vi "autonomousbarrystyle.vi"() -> ()   [LabVIEW 2010, in "Rampage.lvrbt"]
uses:
  Rampage.lvrbt
  <vilib>/NXT/Dual Mode Library/Waits/Wait_Num(msec).vi
  <vilib>/NXT/Block Support/NXT_InputPort.ctl
  <vilib>/NXT/HiTechnic/HiTechnic Controls/HiTechnic Port.ctl
  <vilib>/NXT/Subs/MotorOutput.ctl
  <vilib>/NXT/Subs/MotorXNode.DC Motor Type.ctl
  <vilib>/NXT/Subs/MotorXNode.2DCMotor.ctl
  <vilib>/NXT/Subs/LVHSConnector.ctl
  <vilib>/NXT/NXTIO Xnodes/NXTIONodeSubVIs/TETRIX IO Move DC Motors.vi
  <vilib>/NXT/NXTIO Xnodes/NXTIOXNode/NXTIO.xnode
  <vilib>/NXT/Dual Mode Library/Motors/MotorOn.vi
  <vilib>/NXT/Dual Mode Library/prims/inRangeAndCoerce/inRangeAndCoerce_int.vi
  <vilib>/NXT/NXTIO Xnodes/NXTIONodeSubVIs/TETRIX IO Stop DC Motors.vi
  <vilib>/NXT/NXTIO Xnodes/AddressXNode/NXTIOAddress.xnode
  <vilib>/NXT/Dual Mode Library/Sensors/Sonar_cm.vi
  <vilib>/NXT/Dual Mode Library/Waits/Wait_Num.vi
panel:
  out "Enabled":bool
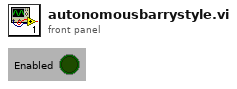
[diagram p1: front panel]
types:
  T1 = typedef "LVHSConnector.ctl" = cluster{"Hardware":string, "Flattened String":string}
  T2 = typedef "MotorOutput.ctl" = u8
  T3 = typedef "MotorXNode.DC Motor Type.ctl" = enum16{"DC Motor"}
  T4 = cluster{"DC Motor":T3, "Address":i16, "Address":i16}
  T5 = typedef "HiTechnic Port.ctl" = cluster{"Port":T6, "MUX Port":u8}
  T6 = typedef "NXT_InputPort.ctl" = u8
  T7 = cluster{"Direction (0-9)":i16, "Signal Strength (Array)":u8[]}
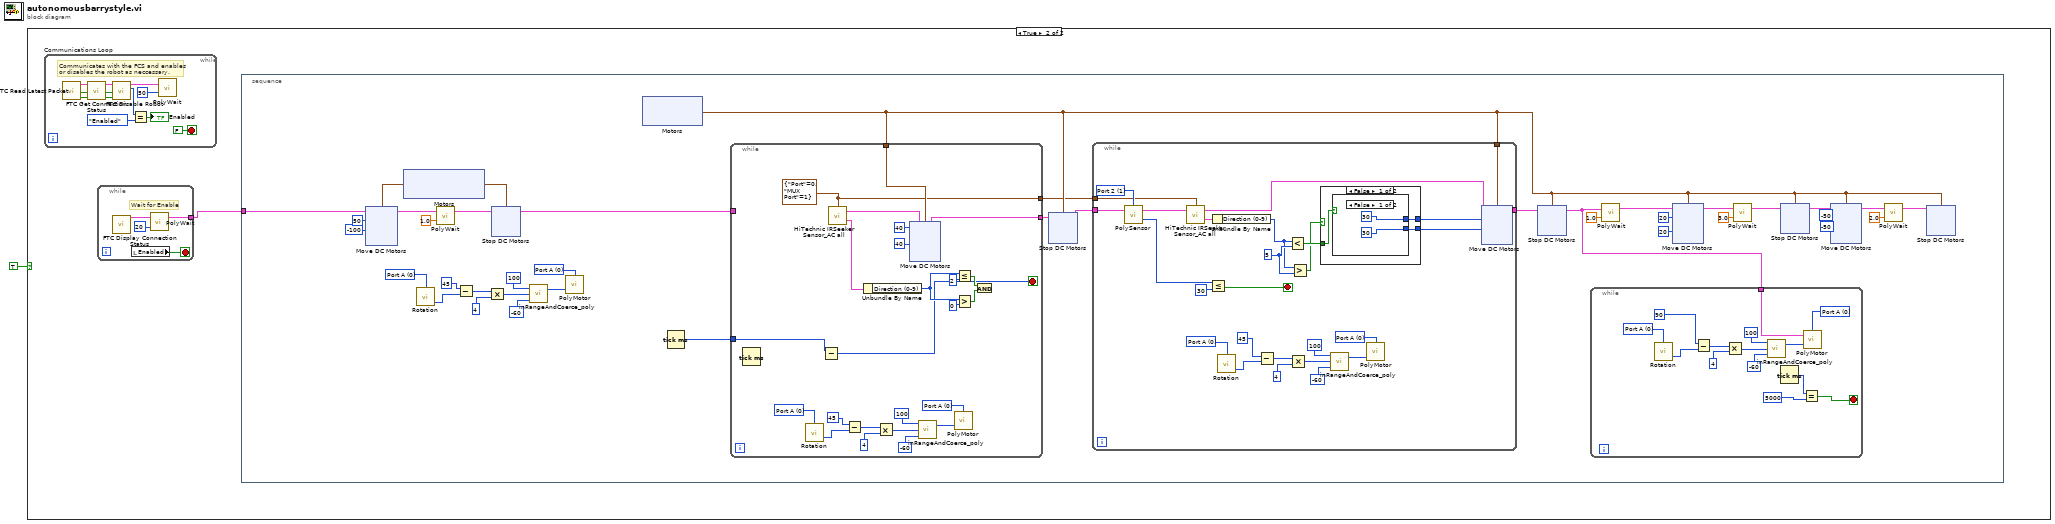
[diagram p0: block diagram]
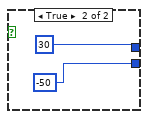
[diagram p3: hidden frame]
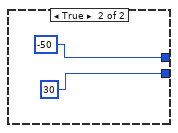
[diagram p4: hidden frame]
diagram:
  n1 = case shown="True" TRUE {
    frame False {
    }
    frame True {
      n2 = while "Communications Loop" {
        stop <- FALSE stop-if-true
        # "Communicates with the FCS and enables \nor disables the robot as neccessary."
        n3 = call <vilib>:"FTC Read Latest Packet.vi"() -> ("Packet Received?"=w216:bool, "Stopped?"=w215:bool, "NXT"=w218:T1)  [unwired: 6 in, 3 out]
        n4 = call <vilib>:"FTC Get Connection Status.vi"("Packet Received?"=w216, "Stopped?"=w215, "NXT"=w218) -> ("Online?"=w207:bool, "Stopped?"=w208:bool, "NXT"=w217:T1)  [unwired: 5 in]
        n5 = call <vilib>:"FTC Disable Robot.vi"("Online?"=w207, "Stopped?"=w208, "NXT"=w217) -> ("Enabled?"=w211:enum16{"Disabled", "Enabled"}, "NXT"=w213:T1)  [unwired: 3 in]
        n6 = Equal?(x=w211, y=enum16{"Disabled", "Enabled"}."Enabled") -> (x = y?=→"Enabled":bool)
        n7 = call-poly <vilib>:"PolyWait.vi"("Time (100 msec)"=u32 50 ("Time (msec)"), "NXT"=w213) -> ()  [unwired: 2 in, 1 out]
      }
      n8 = while {
        tunnel: [w204] -> w2
        stop <- w205 stop-if-true
        # "Wait for Enable"
        n9 = call <vilib>:"FTC Display Connection Status.vi"() -> ("NXT"=w203:T1)  [unwired: 11 in]
        n10 = local read "Enabled"() -> (w205:bool)
        n11 = call-poly <vilib>:"PolyWait.vi"("Time (100 msec)"=u32 20 ("Time (msec)"), "NXT"=w203) -> ("NXT"=w204:T1)  [unwired: 2 in]
      }
      n12 = stacked-sequence {
        tunnel: w2 -> [w5]
        frame #0 {
          w32 = T2 0 items=["Port A"=0, "Port B"=1, "Port C"=2, "Ports A & B"=4, "Ports A & C"=5, "Ports B & C"=6, "All Ports"=3] ("Output Port (All Ports)")
          w30 = u8 0 items=["Port A", "Port B", "Port C"] ("Port (Port A)")
          n13 = xnode "Motors"() -> ("DC Motor"=w40:T4)
          n14 = xnode "Move DC Motors"("Power/Speed 1"=i8 50, "Motors"=w40, "NXT"=w5, "Power/Speed 2"=i8 -100) -> ("NXT"=w38:T1)
          n15 = call <vilib>:"Rotation.vi"("Port (Port A)"=w30) -> ("Angle of Rotation"=w33:i32)  [unwired: 2 in, 1 out]
          n16 = call-poly <vilib>:"PolyWait.vi"("Time (1 sec)"=sgl 1.0, "NXT"=w38) -> ("NXT"=w35:T1)  [unwired: 2 in]
          n17 = Subtract(x=45 ("Claw\nPosition"), y=w33) -> (x-y=w31:i32)
          n18 = Multiply(x=w31, y=4) -> (x*y=w29:i32)
          n19 = xnode "Stop DC Motors"("Motors"=w40, "NXT"=w35) -> ("NXT"=w21:T1)
          n20 = call-poly <vilib>:"inRangeAndCoerce_poly.vi"("lower limit"=-60, "x"=w29, "upper limit"=100) -> ("coerced(x)"=w26:i32)  [unwired: 1 out]
          n21 = call-poly <vilib>:"PolyMotor.vi"("Power (75)"=w26, "Output Port (All Ports)"=w32) -> ()  [unwired: 2 in, 1 out]
          n22 = xnode "Motors"() -> ("DC Motor"=w23:T4)
          n23 = Tick Count (ms)() -> (millisecond timer value=w3:u32)
          n24 = while {
            tunnel: [w191] -> w9
            tunnel: w23 -> [w188]
            tunnel: [w175] -> w4
            tunnel: w21 -> [_]
            tunnel: w3 -> [w170]
            stop <- w169 stop-if-true
            w180 = T2 0 items=["Port A"=0, "Port B"=1, "Port C"=2, "Ports A & B"=4, "Ports A & C"=5, "Ports B & C"=6, "All Ports"=3] ("Output Port (All Ports)")
            w182 = u8 0 items=["Port A", "Port B", "Port C"] ("Port (Port A)")
            w175 = T5 {"Port"=0, "MUX Port"=1} ("Port/MUX")
            n25 = Tick Count (ms)() -> ()  [unwired: 1 out]
            n26 = call <vilib>:"Rotation.vi"("Port (Port A)"=w182) -> ("Angle of Rotation"=w179:i32)  [unwired: 2 in, 1 out]
            n27 = Subtract(x=w170) -> (y=w168:u32, x-y=w169:u32)
            n28 = call <vilib>:"HiTechnic IRSeeker Sensor_AC all.vi"("Port/MUX"=w175) -> ("All Info"=w176:T7, "NXT"=w192:T1)  [unwired: 2 in]
            n29 = Subtract(x=45 ("Claw\nPosition"), y=w179) -> (x-y=w181:i32)
            n30 = Unbundle By Name(w176) -> ("Direction (0-9)"=w173:i16)
            n31 = Multiply(x=w181, y=4) -> (x*y=w183:i32)
            n32 = xnode "Move DC Motors"("Power/Speed 2"=i8 40, "Power/Speed 1"=i8 40, "Motors"=w188, "NXT"=w192) -> ("NXT"=w191:T1)
            n33 = call-poly <vilib>:"inRangeAndCoerce_poly.vi"("lower limit"=-60, "x"=w183, "upper limit"=100) -> ("coerced(x)"=w186:i32)  [unwired: 1 out]
            n34 = call-poly <vilib>:"PolyMotor.vi"("Power (75)"=w186, "Output Port (All Ports)"=w180) -> ()  [unwired: 2 in, 1 out]
            n35 = Less Or Equal?(x=w173, y=i16 2) -> (x <= y?=w172:bool)
            n36 = Greater?(x=w173, y=i16 0) -> (0:w171:bool)
            n37 = And(x=w172, y=w171) -> ()  [unwired: 1 out]
          }
          n38 = xnode "Stop DC Motors"("Motors"=w23, "NXT"=w9) -> ("NXT"=w24:T1)
          n39 = while {
            tunnel: [w139] -> w8
            tunnel: w23 -> [w138]
            tunnel: w24 -> [w116]
            tunnel: w4 -> [w114]
            stop <- w115 stop-if-true
            w119 = T2 0 items=["Port A"=0, "Port B"=1, "Port C"=2, "Ports A & B"=4, "Ports A & C"=5, "Ports B & C"=6, "All Ports"=3] ("Output Port (All Ports)")
            w121 = u8 0 items=["Port A", "Port B", "Port C"] ("Port (Port A)")
            w130 = i16 5 ("y")
            w136 = T6 1 items=["Port 1", "Port 2", "Port 3", "Port 4"] ("Port (Port 4)")
            n40 = call-poly <vilib>:"PolySensor.vi"("NXT"=w116, "Port (Port 4)"=w136) -> ("Distance (cm)"=w137:i16, "NXT"=w135:T1)  [unwired: 1 in]
            n41 = call <vilib>:"HiTechnic IRSeeker Sensor_AC all.vi"("NXT"=w135, "Port/MUX"=w114) -> ("All Info"=w134:T7, "NXT"=w133:T1)  [unwired: 1 in]
            n42 = Less Or Equal?(x=w137, y=i16 30) -> (x <= y?=w115:bool)
            n43 = Unbundle By Name(w134) -> ("Direction (0-9)"=w129:i16)
            n44 = call <vilib>:"Rotation.vi"("Port (Port A)"=w121) -> ("Angle of Rotation"=w118:i32)  [unwired: 2 in, 1 out]
            n45 = Subtract(x=45 ("Claw\nPosition"), y=w118) -> (x-y=w120:i32)
            n46 = Less?(x=w129, y=w130) -> (x < y?=w128:bool)
            n47 = Multiply(x=w120, y=4) -> (x*y=w122:i32)
            n48 = Greater?(x=w129, y=w130) -> (0:w127:bool)
            n49 = case shown="False" w127 {
              tunnel: [w143 i8 -50 ("Power/Speed 2")] -> w132
              tunnel: [w142 i8 30 ("Power/Speed 1")] -> w131
              tunnel: w128 -> [w141 _]
              frame False {
                n50 = case shown="False" w141 {
                  tunnel: [i8 30 ("Power/Speed 1") i8 30 ("Power/Speed 2")] -> w143
                  tunnel: [i8 30 ("Power/Speed 2") i8 -50 ("Power/Speed 1")] -> w142
                  frame False {
                  }
                  frame True {
                  }
                }
              }
              frame True {
              }
            }
            n51 = call-poly <vilib>:"inRangeAndCoerce_poly.vi"("lower limit"=-60, "x"=w122, "upper limit"=100) -> ("coerced(x)"=w125:i32)  [unwired: 1 out]
            n52 = call-poly <vilib>:"PolyMotor.vi"("Power (75)"=w125, "Output Port (All Ports)"=w119) -> ()  [unwired: 2 in, 1 out]
            n53 = xnode "Move DC Motors"("Power/Speed 2"=w131, "Power/Speed 1"=w132, "Motors"=w138, "NXT"=w133) -> ("NXT"=w139:T1)
          }
          n54 = xnode "Stop DC Motors"("Motors"=w23, "NXT"=w8) -> ("NXT"=w22:T1)
          n55 = while {
            tunnel: w22 -> [w63]
            stop <- w60 stop-if-true
            w65 = T2 0 items=["Port A"=0, "Port B"=1, "Port C"=2, "Ports A & B"=4, "Ports A & C"=5, "Ports B & C"=6, "All Ports"=3] ("Output Port (All Ports)")
            w67 = u8 0 items=["Port A", "Port B", "Port C"] ("Port (Port A)")
            n56 = call <vilib>:"Rotation.vi"("Port (Port A)"=w67) -> ("Angle of Rotation"=w64:i32)  [unwired: 2 in, 1 out]
            n57 = Subtract(x=90 ("Claw\nPosition"), y=w64) -> (x-y=w66:i32)
            n58 = Multiply(x=w66, y=4) -> (x*y=w68:i32)
            n59 = call-poly <vilib>:"inRangeAndCoerce_poly.vi"("lower limit"=-60, "x"=w68, "upper limit"=100) -> ("coerced(x)"=w71:i32)  [unwired: 1 out]
            n60 = Tick Count (ms)() -> (millisecond timer value=w62:u32)
            n61 = Equal?(x=w62, y=u32 5000) -> (x = y?=w60:bool)
            n62 = call-poly <vilib>:"PolyMotor.vi"("Power (75)"=w71, "NXT"=w63, "Output Port (All Ports)"=w65) -> ()  [unwired: 1 in, 1 out]
          }
          n63 = call-poly <vilib>:"PolyWait.vi"("Time (1 sec)"=sgl 1.0, "NXT"=w22) -> ("NXT"=w20:T1)  [unwired: 2 in]
          n64 = xnode "Move DC Motors"("Power/Speed 2"=i8 20, "Power/Speed 1"=i8 20, "Motors"=w23, "NXT"=w20) -> ("NXT"=w12:T1)
          n65 = call-poly <vilib>:"PolyWait.vi"("Time (1 sec)"=sgl 3.0, "NXT"=w12) -> ("NXT"=w14:T1)  [unwired: 2 in]
          n66 = xnode "Stop DC Motors"("Motors"=w23, "NXT"=w14) -> ("NXT"=w15:T1)
          n67 = xnode "Move DC Motors"("Power/Speed 2"=i8 -50, "Power/Speed 1"=i8 -50, "Motors"=w23, "NXT"=w15) -> ("NXT"=w7:T1)
          n68 = call-poly <vilib>:"PolyWait.vi"("Time (1 sec)"=sgl 2.0, "NXT"=w7) -> ("NXT"=w16:T1)  [unwired: 2 in]
          n69 = xnode "Stop DC Motors"("Motors"=w23, "NXT"=w16) -> ()  [unwired: 1 out]
        }
      }
    }
  }
